vi "Speed Benchmark.vi"() -> ()   [LabVIEW 2015]
uses:
  <vilib>/FPGAPlugInAG/cRIO-9030/niLvFpga_Open_cRIO-9030.vi
  <vilib>/rvi/interface/common/dynamic/niFpgaDynamicAddResources.vi
  <vilib>/FPGAPlugInAG/Dynamic/niLvFpga_Reset_Dynamic.vi
  <vilib>/FPGAPlugInAG/Dynamic/niLvFpga_Run_Dynamic.vi
  <vilib>/Utility/error.llb/Error Cluster From Error Code.vi
  <vilib>/rvi/errors/niLvFpgaAdjustHostInterfaceError.vi
  <vilib>/rvi/interface/nirviOpenFPGA/nirviOpenFPGA.xnode
  FPGA Bitfiles/BELKINEAGLE_FPGATarget_SpeedBenchmark_496QbYhWNkg.lvbitx
  <vilib>/rvi/interface/nirviMethod/nirviMethod.xnode
  <vilib>/rvi/interface/nirviReadWriteControl/nirviReadWriteControl.xnode
  <vilib>/rvi/errors/niLvFpgaMergeErrorWithErrorCode.vi
  <vilib>/FPGAPlugInAG/Dynamic/niLvFpga_ConfigureFifo_Dynamic.vi
  <vilib>/FPGAPlugInAG/Dynamic/niLvFpga_StartFifo_Dynamic.vi
  NiFpgaLv.dll
  <vilib>/rvi/interface/Simulation/niFpgaSimulationCallBeginRW.vi
  <vilib>/FPGAPlugInAG/Dynamic/niLvFpga_StopFifo_Dynamic.vi
  <vilib>/FPGAPlugInAG/Dynamic/niLvFpga_WriteFifo_Dynamic.vi
panel:
  out "Write Interval":u32
  out "Last index":i32
  out "First index":u32
  out "elements counter":u32
  out "error out":errorcluster
  out "TicksOut":u32
  in  "reset":bool
  in  "stop":bool
  in  "send":bool
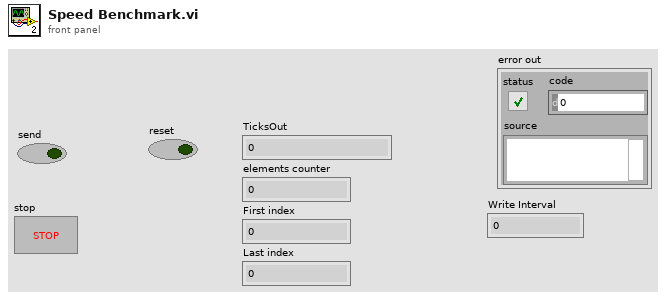
[diagram p1: front panel]
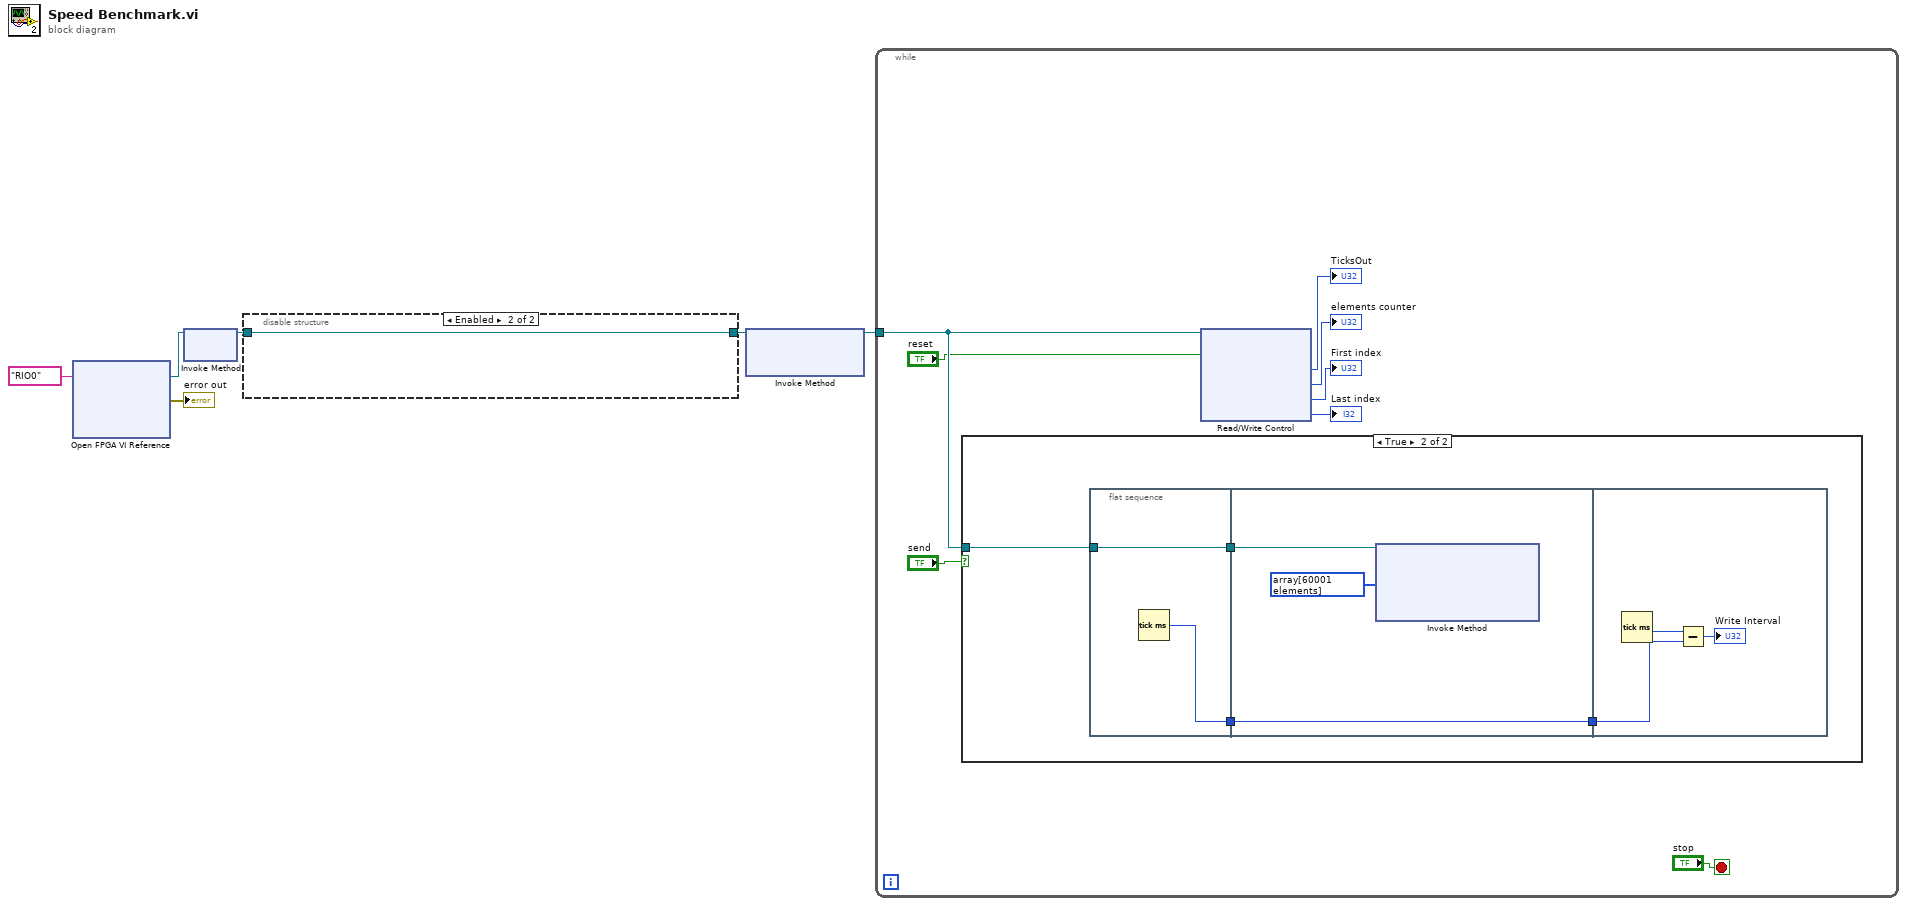
[diagram p0: block diagram]
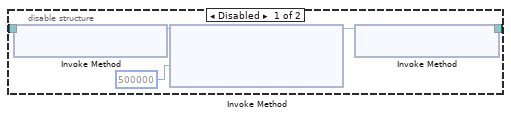
[diagram p2: hidden frame]
diagram:
  n1 = xnode "Open FPGA VI Reference"("resource name"=tag "RIO0") -> ("FPGA VI Reference Out"=w4:refnum<k20>, "error out"=→"error out":errorcluster)  [unwired: 1 in]
  n2 = xnode "Invoke Method"("FPGA VI Reference In"=w4) -> ("FPGA VI Reference Out"=w3:refnum<k20>)  [unwired: 1 in, 1 out]
  n3 = disable-structure shown="Enabled" {
    disable-tunnel: w3 -> [w8 w12]
    disable-tunnel: [w7 w12] -> w1
    frame Disabled {
      n4 = xnode "Invoke Method"("FPGA VI Reference In"=w8) -> ("FPGA VI Reference Out"=w11:refnum<k20>)  [unwired: 1 in, 1 out]
      n5 = xnode "Invoke Method"("FPGA VI Reference In"=w11, "Requested Depth"=u32 500000) -> ("FPGA VI Reference Out"=w10:refnum<k20>)  [unwired: 1 in, 2 out]
      n6 = xnode "Invoke Method"("FPGA VI Reference In"=w10) -> ("FPGA VI Reference Out"=w7:refnum<k20>)  [unwired: 1 in, 1 out]
    }
    frame Enabled {
    }
  }
  n7 = xnode "Invoke Method"("FPGA VI Reference In"=w1) -> ("FPGA VI Reference Out"=w2:refnum<k20>)  [unwired: 2 in, 1 out]
  n8 = while {
    tunnel: w2 -> [w14]
    stop <- "stop" stop-if-true
    n9 = case shown="True" "send" {
      tunnel: w14 -> [_ w24]
      frame False {
      }
      frame True {
        n10 = flat-sequence {
          tunnel: w24 -> [w26]
          tunnel: [w26] -> w23
          tunnel: [w25] -> w22
          tunnel: w23 -> [w29]
          tunnel: w22 -> [w27]
          tunnel: [w27] -> w21
          tunnel: w21 -> [w31]
          frame #0 {
            n11 = Tick Count (ms)() -> (millisecond timer value=w25:u32)
          }
          frame #1 {
            n12 = xnode "Invoke Method"("FPGA VI Reference In"=w29, "Data"=u8[] array[60001 elements]) -> ()  [unwired: 2 in, 3 out]
          }
          frame #2 {
            n13 = Tick Count (ms)() -> (millisecond timer value=w32:u32)
            n14 = Subtract(x=w32, y=w31) -> (x-y=→"Write Interval":u32)
          }
        }
      }
    }
    n15 = xnode "Read/Write Control"("FPGA VI Reference In"=w14, "reset"="reset") -> ("TicksOut"=→"TicksOut":u32, "elements counter"=→"elements counter":u32, "First index"=→"First index":u32, "Last index"=→"Last index":i32)  [unwired: 1 in, 2 out]
  }
